vi "Update DIs in MeasDataQ.vi"(8 "error in (no error)":errorcluster, 9 "TimeStamp":timestamp, 10 "LP2":bool, 11 "LP1":bool) -> (0 "error out":errorcluster, 3 "orData out":T1)   [LabVIEW 2020]
doc: "Developed by Kevin Thompson\nThompson Engineering, LLC\nkevin@thompsonengineering.net"
uses:
  TD MeasData QRef.ctl
  TD MeasData--cluster.ctl
  GBL DataQ Ref.vi
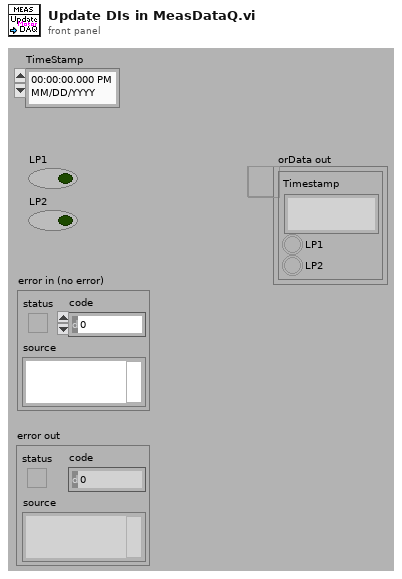
[diagram p1: front panel]
types:
  T1 = typedef "TD MeasData QRef.ctl" = refnum<queue>
  T2 = typedef "TD MeasData--cluster.ctl" = cluster{"Timestamp":timestamp, "LP1":bool, "LP2":bool}
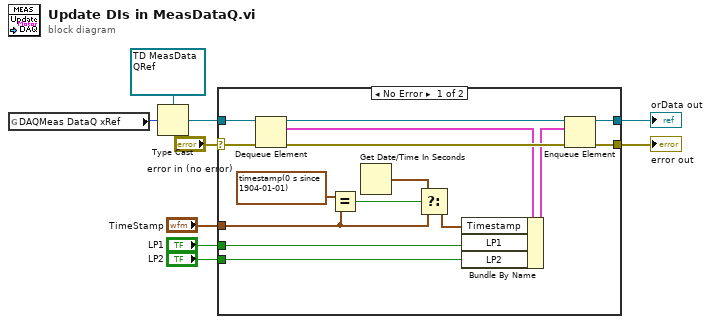
[diagram p0: block diagram]
diagram:
  n1 = global read "GBL DataQ Ref.vi" "DAQMeas DataQ xRef"() -> (w3:u32)
  n2 = Type Cast(type=T1 refnum ("orData in"), x=w3) -> (*(type *) &x=w5:T1)
  n3 = case shown="No Error" "error in (no error)" {
    selector: "error in (no error)" -> [w19 w25]
    tunnel: w5 -> [w24 w26]
    tunnel: [w21 w25] -> w9
    tunnel: [w20 w26] -> w8
    tunnel: "TimeStamp" -> [w14 _]
    tunnel: "LP2" -> [w11 _]
    tunnel: "LP1" -> [w10 _]
    frame No Error {
      n4 = Dequeue Element(queue=w24, error in (no error)=w19) -> (queue out=w22:T1, element=w18:T2, error out=w23:errorcluster)  [unwired: 1 in, 1 out]
      n5 = Equal?(x=timestamp(0 s since 1904-01-01) ("TimeStamp"), y=w14) -> (x = y?=w15:bool)
      n6 = Get Date/Time In Seconds() -> (seconds since 1Jan1904=w12:timestamp)
      n7 = Select(t=w12, s=w15, f=w14) -> (s? t:f=w13:timestamp)
      n8 = Bundle By Name(cluster=w18, "Timestamp"=w13, "LP1"=w10, "LP2"=w11) -> (w17:T2)
      n9 = Enqueue Element(queue=w22, element=w17, error in (no error)=w23) -> (queue out=w20:T1, error out=w21:errorcluster)  [unwired: 1 in, 1 out]
    }
    frame Error {
    }
  }
  "orData out" <- w8
  "error out" <- w9
